vi "fgt set pressure Response.vi"(8 "error in (no error)":errorcluster, 10 "value":u8, 11 "pressureIndex":u32) -> (0 "error out":errorcluster)   [LabVIEW 2020, in "fgt_SDK.lvlib"]
doc: "Set pressure controller response. This function can be used to customise response time for your set-up.\nFor FlowEZ available values are 0: use of fast switch vales or 1: do not use fast switch vales. Default value is 0.\nFor MFCS available values are from 1 to 255. Higher the value, longer is the response time. Default value is 5."
uses:
  fgt_SDK.lvlib
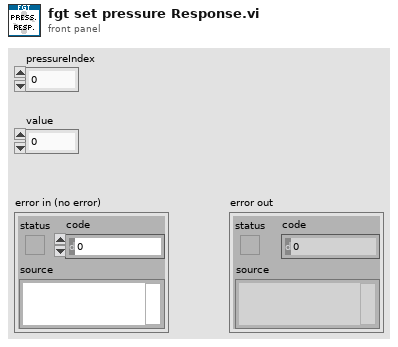
[diagram p1: front panel]
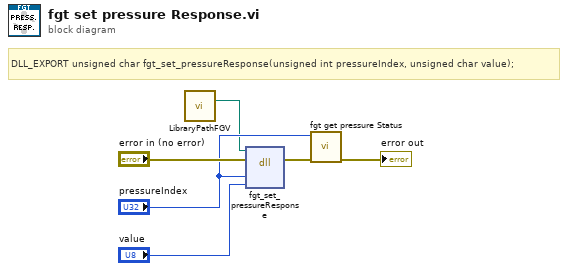
[diagram p0: block diagram]
diagram:
  # "DLL_EXPORT unsigned char fgt_set_pressureResponse(unsigned int pressureIndex, unsigned char value);"
  n1 = call "LibraryPathFGV.vi"() -> ("Path Out"=w1:path)  [unwired: 14 in, 1 out]
  n2 = dll-call lib="C:/Workspace/fgt-SDK/LabVIEW/dlls/fgt_SDK_*.*" fn="fgt_set_pressureResponse"(path in=w1, error in="error in (no error)", "pressureIndex"="pressureIndex", "value"="value") -> (error out=w4:errorcluster)  [unwired: 4 in, 1 out]
  n3 = call "fgt get pressure Status.vi"("error in (no error)"=w4, "pressureIndex"="pressureIndex") -> ("error out"=→"error out":errorcluster)  [unwired: 9 in]
